vi "Convert Unit Data.vi"(0 "VISA resource name":refnum<visa-resource-name>, 7 "Unit Data (\"\")":string, 11 "error in (no error)":errorcluster) -> (4 "VISA resource name out":refnum<visa-resource-name>, 6 "Channel":string[](array[string]), 8 "Unit":string[](array[string]), 10 "Data Status":i32[](array[ring]) items=["Normal", "Differential Input", "Skip"], 14 "Decimal Position":i32[](array[numeric]) max=4 step=1, 15 "error out":errorcluster)   [LabVIEW 2020, in "Yokogawa GX Series.lvlib"]
doc: "This VI converts unit data to 4 parts, which are channel number, data status, decimal position, and unit."
uses:
  <instrlib>/Yokogawa GX Series/Yokogawa GX Series.lvlib
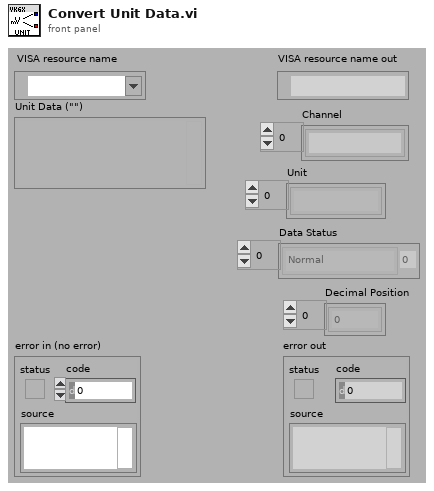
[diagram p1: front panel]
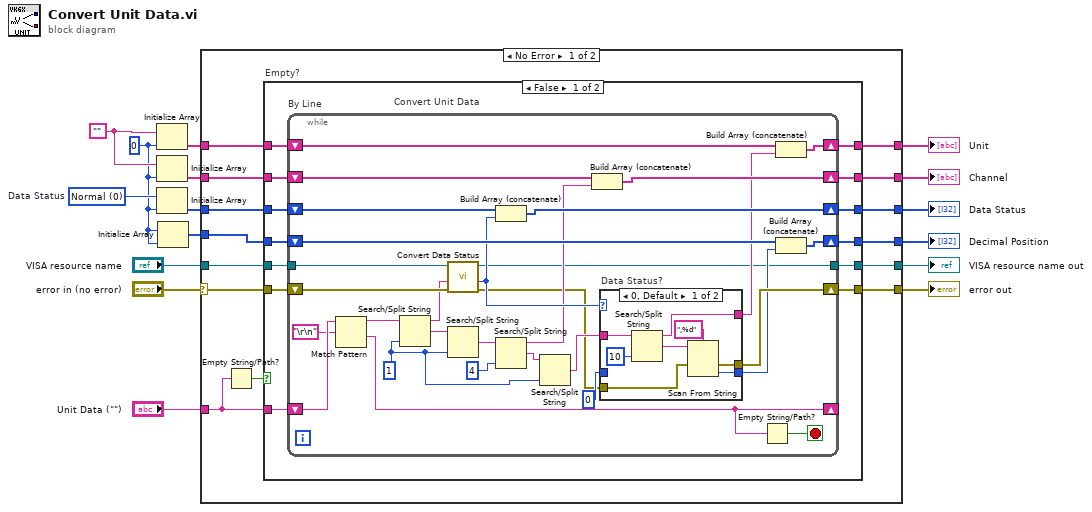
[diagram p0: block diagram]
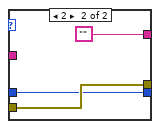
[diagram p2: hidden frame]
diagram:
  w6 = 0 items=["Normal", "Differential Input", "Skip"]  # Data Status
  w4 = ""
  w2 = 0
  n1 = Initialize Array(w4, w2) -> (w15:string[])
  n2 = Initialize Array(w4, w2) -> (w5:string[])
  n3 = Initialize Array(w6, w2) -> (w14:i32[])
  n4 = Initialize Array(w2, w2) -> (w3:i32[])
  n5 = case shown="No Error" "error in (no error)" {
    selector: "error in (no error)" -> [w17 w91]
    tunnel: "VISA resource name" -> [w30 w92]
    tunnel: w15 -> [w29 w96]
    tunnel: w14 -> [w28 w94]
    tunnel: "Unit Data (\"\")" -> [w26 _]
    tunnel: [w25 w96] -> w12
    tunnel: [w24 w94] -> w11
    tunnel: [w23 w95] -> w10
    tunnel: [w22 w93] -> w9
    tunnel: [w21 w91] -> w8
    tunnel: [w20 w92] -> w7
    tunnel: w5 -> [w19 w95]
    tunnel: w3 -> [w18 w93]
    frame No Error {
      n6 = Empty String/Path?(string/path=w26) -> (empty?=w27:bool)
      n7 = case "Empty?" shown="False" w27 {
        tunnel: w19 -> [w31 w85]
        tunnel: w26 -> [w43 _]
        tunnel: w17 -> [w42 w88]
        tunnel: [w41 w88] -> w21
        tunnel: [w40 w86] -> w22
        tunnel: w30 -> [w39 w89]
        tunnel: [w38 w89] -> w20
        tunnel: w28 -> [w37 w87]
        tunnel: [w36 w85] -> w23
        tunnel: [w35 w90] -> w25
        tunnel: w18 -> [w32 w86]
        tunnel: w29 -> [w34 w90]
        tunnel: [w33 w87] -> w24
        frame False {
          # "Convert Unit Data"
          n8 = while "By Line" {
            shift-left: w32 -> [w61]
            shift-right: [w60] -> w40
            shift-left: w42 -> [w52]
            shift-right: [w62] -> w41
            shift-left: w34 -> [w58]
            shift-right: [w56] -> w35
            shift-left: w31 -> [w69]
            shift-right: [w68] -> w36
            shift-left: w37 -> [w70]
            shift-right: [w67] -> w33
            shift-left: w43 -> [w72]
            shift-right: [w73] -> _
            tunnel: w39 -> [w53]
            tunnel: [w45] -> w38
            stop <- w55 stop-if-true
            w49 = 1
            n9 = Match Pattern(string=w72, regular expression="\r\n") -> (before substring=w66:string, after substring=w73:string)  [unwired: 3 out]
            n10 = Search/Split String(string=w66, offset (0)=w49) -> (substring before match=w51:string, match + rest of string=w64:string)  [unwired: 2 out]
            n11 = call <instrlib>:"Convert Data Status.vi"("error in (no error)"=w52, "Data Status String (\"\")"=w51, "VISA resource name"=w53) -> ("error out"=w44:errorcluster, "Data Status"=w50:i32, "VISA resource name out"=w45:refnum<visa-resource-name>)  [unwired: 6 out]
            n12 = Search/Split String(string=w64, offset (0)=w49) -> (match + rest of string=w63:string)  [unwired: 3 out]
            n13 = Build Array (concatenate)(w70, w50) -> (w67:i32[])
            n14 = Search/Split String(string=w63, offset (0)=4) -> (substring before match=w46:string, match + rest of string=w48:string)  [unwired: 2 out]
            n15 = Search/Split String(string=w48, offset (0)=w49) -> (match + rest of string=w47:string)  [unwired: 1 in, 2 out]
            n16 = Build Array (concatenate)(w69, w46) -> (w68:string[])
            n17 = case "Data Status?" shown="0, Default" w50 {
              tunnel: w44 -> [w81 w84]
              tunnel: [w80 w84] -> w62
              tunnel: w47 -> [w77 _]
              tunnel: [w76 w83] -> w59
              tunnel: [w75 ""] -> w57
              tunnel: 0 -> [_ w83]
              frame 0, Default {
                n18 = Search/Split String(string=w77, offset (0)=10) -> (substring before match=w75:string, match + rest of string=w74:string)  [unwired: 2 out]
                n19 = Scan From String(format string=",%d", input string=w74, error in=w81) -> (error out=w80:errorcluster, output 1=w76:i32)  [unwired: 1 in, 3 out]
              }
              frame 2 {
              }
            }
            n20 = Empty String/Path?(string/path=w73) -> (empty?=w55:bool)
            n21 = Build Array (concatenate)(w58, w57) -> (w56:string[])
            n22 = Build Array (concatenate)(w61, w59) -> (w60:i32[])
          }
        }
        frame True {
        }
      }
    }
    frame Error {
    }
  }
  "error out" <- w8
  "VISA resource name out" <- w7
  "Unit" <- w12
  "Data Status" <- w11
  "Channel" <- w10
  "Decimal Position" <- w9
